vi "PicoScope4000aGetBlock.vi"(8 "Acquisition Settings":T3 {"Down Sample Ratio" min=1 step=1; "Down-Sample Mode" items=["None", "Aggregate", "Decimate", "Average"]}, 9 "Enabled array":i16[](array[numeric]), 10 "handle in":i16, 11 "error in":errorcluster) -> (0 "Min Buffers":T1, 1 "Buffers (Max or non-aggregated)":T2, 2 "handle out":i16, 3 "error out":errorcluster, 4 "overflow":i16, 6 "noOfSamples":u32)   [LabVIEW 2009]
doc: "This VI collects a block of data from the oscilloscope. This can be called in a loop in order to continually collect blocks of data. The oscilloscope should first be set up by using PicoScope3000aSettings.vi. The VI outputs data arrays in two clusters (max and min). If not using aggregation, 'Min Buffers' is not used."
uses:
  ps4000A.dll
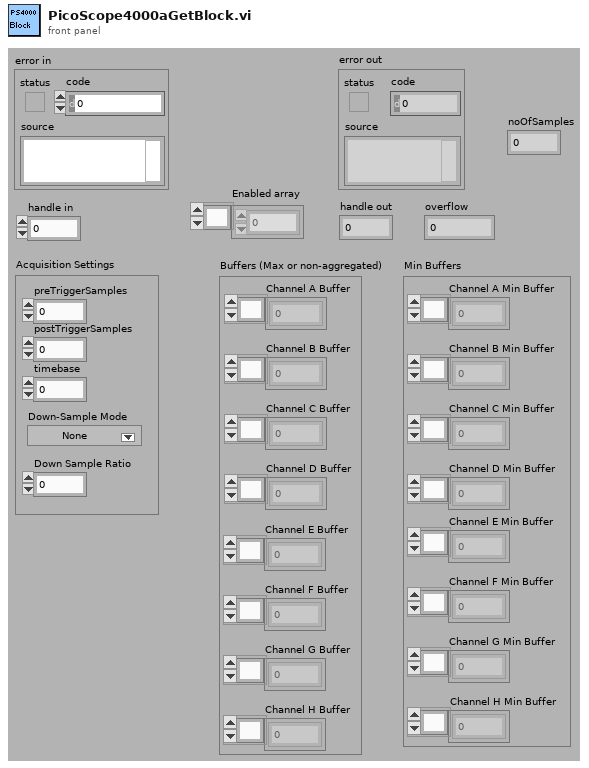
[diagram p1: front panel]
types:
  T1 = cluster{"Channel A Min Buffer":i16[], "Channel B Min Buffer":i16[], "Channel C Min Buffer":i16[], "Channel D Min Buffer":i16[], "Channel E Min Buffer":i16[], "Channel F Min Buffer":i16[], "Channel G Min Buffer":i16[], "Channel H Min Buffer":i16[]}
  T2 = cluster{"Channel D Buffer":i16[], "Channel C Buffer":i16[], "Channel B Buffer":i16[], "Channel A Buffer":i16[], "Channel H Buffer":i16[], "Channel G Buffer":i16[], "Channel F Buffer":i16[], "Channel E Buffer":i16[]}
  T3 = cluster{"preTriggerSamples":i32, "postTriggerSamples":i32, "timebase":u32, "Down-Sample Mode":u32, "Down Sample Ratio":u32}
  T4 = cluster{"Channel A Min Buffer":i16[], "Channel B Min Buffer":i16[], "Channel C Min Buffer":i16[], "Channel D Min Buffer":i16[], "Channel H Min Buffer":i16[], "Channel G Min Buffer":i16[], "Channel F Min Buffer":i16[], "Channel E Min Buffer":i16[]}
  T5 = cluster{"Channel D Buffer":i16[], "Channel C Buffer":i16[], "Channel B Buffer":i16[], "Channel A Buffer":i16[], "Channel E Buffer":i16[], "Channel F Buffer":i16[], "Channel G Buffer":i16[], "Channel H Buffer":i16[]}
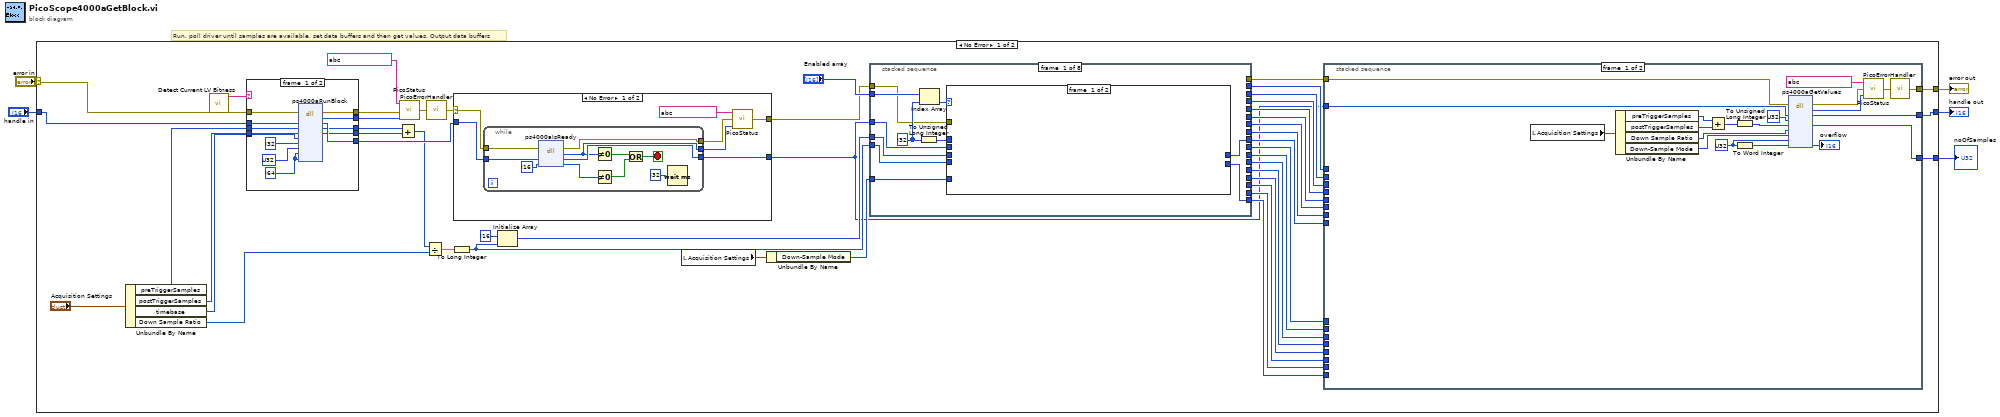
[diagram p0: block diagram]
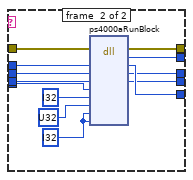
[diagram p2: hidden frame]
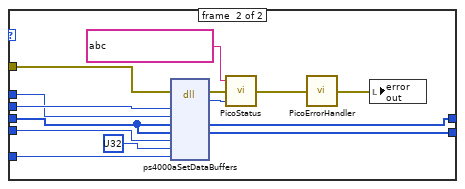
[diagram p3: hidden frame]
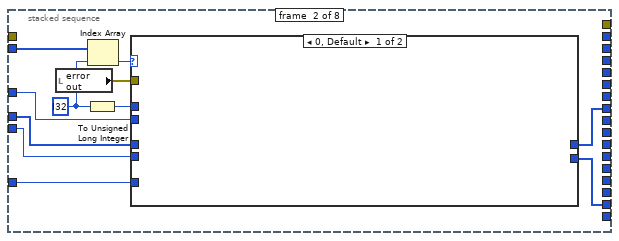
[diagram p4: hidden frame]
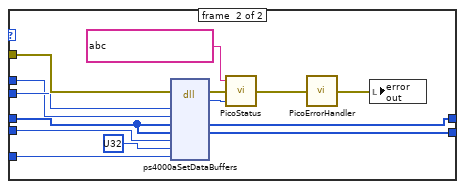
[diagram p5: hidden frame]
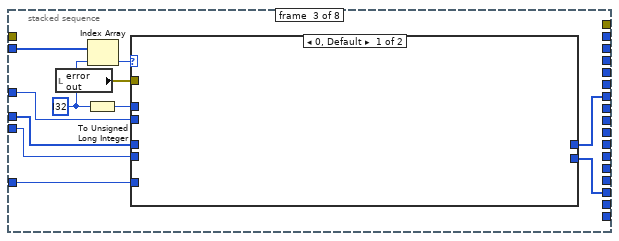
[diagram p6: hidden frame]
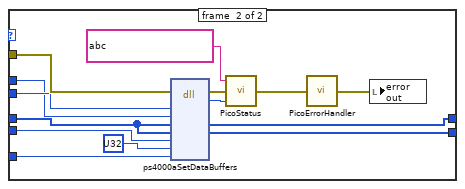
[diagram p7: hidden frame]
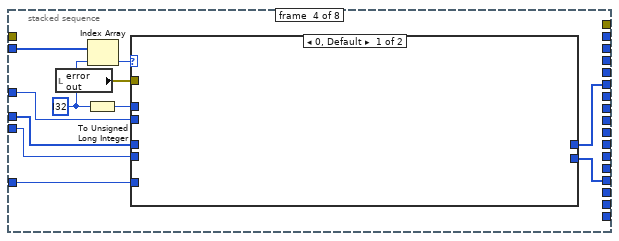
[diagram p8: hidden frame]
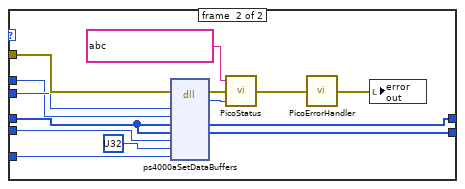
[diagram p9: hidden frame]
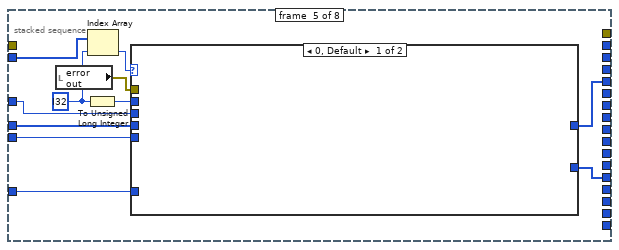
[diagram p10: hidden frame]
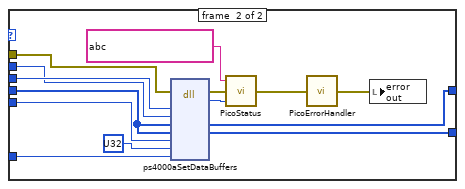
[diagram p11: hidden frame]
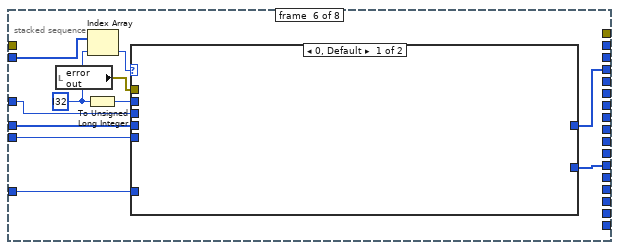
[diagram p12: hidden frame]
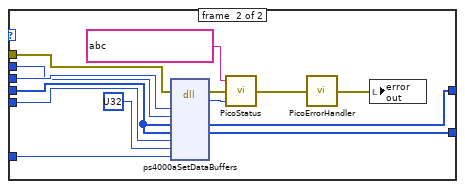
[diagram p13: hidden frame]
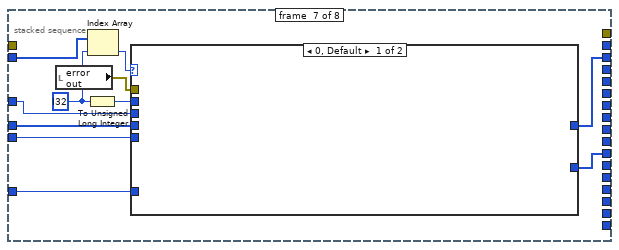
[diagram p14: hidden frame]
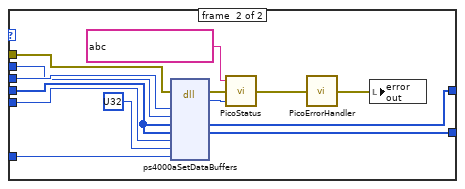
[diagram p15: hidden frame]
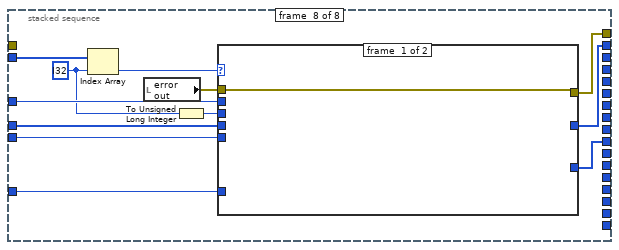
[diagram p16: hidden frame]
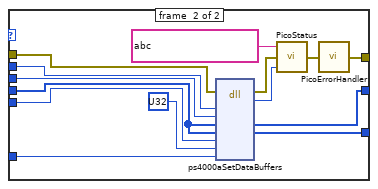
[diagram p17: hidden frame]
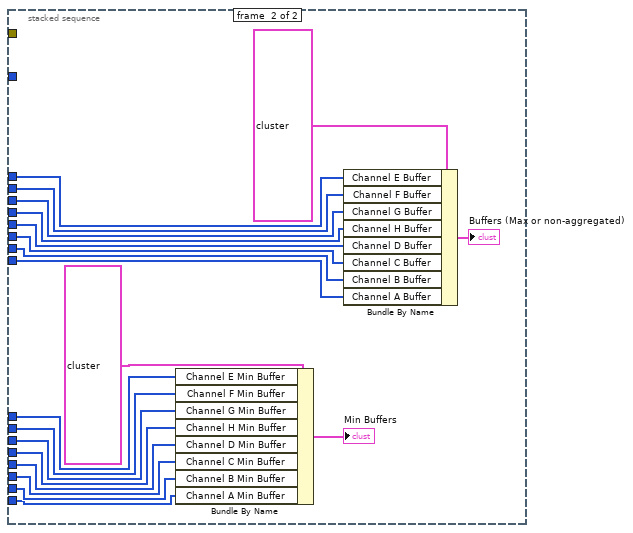
[diagram p18: hidden frame]
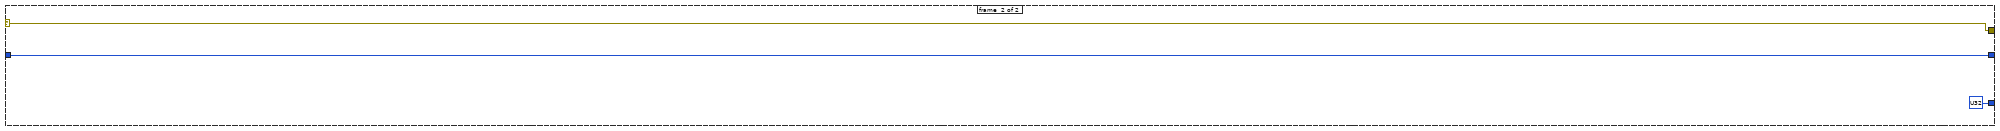
[diagram p20: hidden frame]
diagram:
  # "Run, poll driver until samples are available, set data buffers and then get values. Output data buffers"
  n1 = case shown="No Error" "error in" {
    selector: "error in" -> [w40 w342]
    tunnel: [w41 w342] -> w4
    tunnel: "handle in" -> [w39 w341]
    tunnel: [w38 w341] -> w2
    tunnel: [w7 u32 ? ("noOfSamples")] -> w1
    frame #0 {
      n2 = Unbundle By Name("Acquisition Settings") -> ("preTriggerSamples"=w46:i32, "postTriggerSamples"=w45:i32, "timebase"=w47:u32, "Down Sample Ratio"=w35:u32)
      n3 = call "Detect Current LV Bitness.vi"() -> ("bitness"=w6:string)  [unwired: 11 in]
      n4 = case shown="\"32\", Default" w6 {
        tunnel: [w63 w76] -> w51
        tunnel: [w62 w75] -> w50
        tunnel: [w61 w74] -> w49
        tunnel: w47 -> [w60 w73]
        tunnel: w46 -> [w59 w72]
        tunnel: w45 -> [w58 w71]
        tunnel: [w57 w70] -> w44
        tunnel: [w56 w69] -> w43
        tunnel: w40 -> [w55 w68]
        tunnel: w39 -> [w54 w67]
        frame #0 {
          w53 = i64 ? ("pParameter")
          n5 = dll-call lib="ps4000A.dll" fn="ps4000aRunBlock" ("ps3000.dll:_ps3000_open_unit@0")(error in=w55, "handle"=w54, "preTriggerSamples"=w59, "postTriggerSamples"=w58, "timebase"=w60, "timeindisposed"=i32 ? ("pParameter"), "segmentIndex"=u32 ? ("pParameter"), "lpReady"=w53, "pParameter"=w53) -> (error out=w56:errorcluster, "PICO_STATUS"=w57:u32, "handle"=w63:i16, "preTriggerSamples"=w62:i32, "postTriggerSamples"=w61:i32)  [unwired: 7 in, 1 out]
        }
        frame #1 {
          w65 = i32 ? ("pParameter")
          n6 = dll-call lib="ps4000A.dll" fn="ps4000aRunBlock" ("ps3000.dll:_ps3000_open_unit@0")(error in=w68, "handle"=w67, "preTriggerSamples"=w72, "postTriggerSamples"=w71, "timebase"=w73, "timeindisposed"=i32 ? ("pParameter"), "segmentIndex"=u32 ? ("pParameter"), "lpReady"=w65, "pParameter"=w65) -> (error out=w69:errorcluster, "PICO_STATUS"=w70:u32, "handle"=w76:i16, "preTriggerSamples"=w75:i32, "postTriggerSamples"=w74:i32)  [unwired: 7 in, 1 out]
        }
      }
      n7 = Add(x=w50, y=w49) -> (x+y=w37:i32)
      n8 = call "PicoStatus.vi"("PICO STATUS"=w44, "error in"=w43, "source"=string ?) -> ("error out"=w33:errorcluster)
      n9 = Divide(x=w37, y=w35) -> (x/y=w36:dbl)
      n10 = call "PicoErrorHandler.vi"("error in"=w33) -> ("error out"=w32:errorcluster)
      n11 = To Long Integer(number=w36) -> (32bit integer=w11:i32)
      n12 = case shown="No Error" w32 {
        selector: w32 -> [w324 w338]
        tunnel: w51 -> [w326 w339]
        tunnel: [w325 w339] -> w10
        tunnel: [w323 w338] -> w9
        frame #0 {
          n13 = while {
            tunnel: [w337] -> w325
            tunnel: w326 -> [w336]
            tunnel: [w331] -> w321
            tunnel: w324 -> [w330]
            tunnel: [w329] -> w322
            stop <- w335 stop-if-true
            n14 = dll-call lib="ps4000A.dll" fn="ps4000aIsReady" ("ps3000.dll:_ps3000_open_unit@0")(error in=w330, "handle"=w336, "ready"=i16 ?) -> (error out=w329:errorcluster, "PICO_STATUS"=w331:u32, "handle"=w337:i16, "ready"=w332:i16)  [unwired: 2 in, 1 out]
            n15 = Not Equal To 0?(x=w331) -> (x != 0?=w333:bool)
            n16 = Not Equal To 0?(x=w332) -> (x != 0?=w334:bool)
            n17 = Or(x=w333, y=w334) -> (x .or. y?=w335:bool)
            n18 = Wait (ms)(milliseconds to wait=i32 ?) -> ()  [unwired: 1 out]
          }
          n19 = call "PicoStatus.vi"("PICO STATUS"=w321, "error in"=w322, "source"=string ?) -> ("error out"=w323:errorcluster)
        }
        frame #1 {
        }
      }
      n20 = Initialize Array(i16 ? ("element"), w11) -> (w13:i16[])
      n21 = local read "Acquisition Settings"() -> (w34:T3)
      n22 = Unbundle By Name(w34) -> ("Down-Sample Mode"=w12:u32)
      n23 = stacked-sequence {
        tunnel: [_ _ _ _ _ _ _ w256] -> w30
        tunnel: [_ _ _ _ _ _ w230 _] -> w29
        tunnel: [_ _ _ _ _ w204 _ _] -> w28
        tunnel: [_ _ _ w155 _ _ _ _] -> w27
        tunnel: [_ _ _ _ w180 _ _ _] -> w26
        tunnel: [_ _ w130 _ _ _ _ _] -> w25
        tunnel: [_ w105 _ _ _ _ _ _] -> w24
        tunnel: [w84 _ _ _ _ _ _ _] -> w23
        tunnel: [_ _ _ _ _ _ _ w255] -> w22
        tunnel: [_ _ _ _ _ _ w229 _] -> w21
        tunnel: [_ _ _ _ _ w205 _ _] -> w20
        tunnel: [_ _ _ _ w179 _ _ _] -> w19
        tunnel: [_ _ _ w154 _ _ _ _] -> w18
        tunnel: [_ _ w129 _ _ _ _ _] -> w17
        tunnel: [_ w104 _ _ _ _ _ _] -> w16
        tunnel: [w83 _ _ _ _ _ _ _] -> w15
        tunnel: "Enabled array" -> [w88 w113 w138 w163 w188 w213 w238 w264]
        tunnel: w13 -> [w85 w110 w135 w160 w185 w210 w235 w261]
        tunnel: w9 -> [w78 _ _ _ _ _ _ _]
        tunnel: w10 -> [w86 w111 w136 w161 w186 w211 w236 w262]
        tunnel: w12 -> [w82 w109 w134 w159 w184 w209 w234 w260]
        tunnel: w11 -> [w79 w106 w131 w156 w181 w206 w231 w257]
        tunnel: [_ _ _ _ _ _ _ w254] -> w8
        frame #0 {
          w81 = i32 ? ("index")
          n24 = To Unsigned Long Integer(number=w81) -> (unsigned 32bit integer=w80:u32)
          n25 = Index Array(array=w88, index=w81) -> (element=w87:i16)
          n26 = case shown="1" w87 {
            tunnel: w78 -> [_ w99]
            tunnel: w86 -> [_ w98]
            tunnel: w85 -> [_ w95]
            tunnel: [_ w97] -> w84
            tunnel: [_ w96] -> w83
            tunnel: w82 -> [_ w93]
            tunnel: w80 -> [_ w91]
            tunnel: w79 -> [_ w90]
            frame #0 {
            }
            frame #1 {
              n27 = dll-call lib="ps4000a.dll" fn="ps4000aSetDataBuffers" ("ps3000.dll:_ps3000_open_unit@0")(error in=w99, "handle"=w98, "channel"=w91, "bufferMax"=w95, "bufferMin"=w95, "bufferLth"=w90, "segmentIndex"=u32 ?, "mode"=w93) -> (error out=w102:errorcluster, "PICO_STATUS"=w101:u32, "bufferMax"=w97:i16[], "bufferMin"=w96:i16[])  [unwired: 7 in, 1 out]
              n28 = call "PicoStatus.vi"("PICO STATUS"=w101, "error in"=w102, "source"=string ?) -> ("error out"=w94:errorcluster)
              n29 = call "PicoErrorHandler.vi"("error in"=w94) -> ("error out"=w89:errorcluster)
              n30 = local write "error out"(w89) -> ()
            }
          }
        }
        frame #1 {
          w108 = i32 ? ("index")
          n31 = local read "error out"() -> (w103:errorcluster)
          n32 = To Unsigned Long Integer(number=w108) -> (unsigned 32bit integer=w107:u32)
          n33 = Index Array(array=w113, index=w108) -> (element=w112:i16)
          n34 = case shown="0, Default" w112 {
            tunnel: w103 -> [_ w124]
            tunnel: w111 -> [_ w123]
            tunnel: w110 -> [_ w120]
            tunnel: [_ w122] -> w105
            tunnel: [_ w121] -> w104
            tunnel: w109 -> [_ w114]
            tunnel: w107 -> [_ w117]
            tunnel: w106 -> [_ w116]
            frame #0 {
            }
            frame #1 {
              n35 = dll-call lib="ps4000a.dll" fn="ps4000aSetDataBuffers" ("ps3000.dll:_ps3000_open_unit@0")(error in=w124, "handle"=w123, "channel"=w117, "bufferMax"=w120, "bufferMin"=w120, "bufferLth"=w116, "segmentIndex"=u32 ?, "mode"=w114) -> (error out=w127:errorcluster, "PICO_STATUS"=w126:u32, "bufferMax"=w122:i16[], "bufferMin"=w121:i16[])  [unwired: 7 in, 1 out]
              n36 = call "PicoStatus.vi"("PICO STATUS"=w126, "error in"=w127, "source"=string ?) -> ("error out"=w119:errorcluster)
              n37 = call "PicoErrorHandler.vi"("error in"=w119) -> ("error out"=w115:errorcluster)
              n38 = local write "error out"(w115) -> ()
            }
          }
        }
        frame #2 {
          w133 = i32 ? ("index")
          n39 = local read "error out"() -> (w128:errorcluster)
          n40 = To Unsigned Long Integer(number=w133) -> (unsigned 32bit integer=w132:u32)
          n41 = Index Array(array=w138, index=w133) -> (element=w137:i16)
          n42 = case shown="0, Default" w137 {
            tunnel: w128 -> [_ w149]
            tunnel: w136 -> [_ w148]
            tunnel: w135 -> [_ w145]
            tunnel: [_ w147] -> w130
            tunnel: [_ w146] -> w129
            tunnel: w134 -> [_ w143]
            tunnel: w132 -> [_ w141]
            tunnel: w131 -> [_ w140]
            frame #0 {
            }
            frame #1 {
              n43 = dll-call lib="ps4000a.dll" fn="ps4000aSetDataBuffers" ("ps3000.dll:_ps3000_open_unit@0")(error in=w149, "handle"=w148, "channel"=w141, "bufferMax"=w145, "bufferMin"=w145, "bufferLth"=w140, "segmentIndex"=u32 ?, "mode"=w143) -> (error out=w152:errorcluster, "PICO_STATUS"=w151:u32, "bufferMax"=w147:i16[], "bufferMin"=w146:i16[])  [unwired: 7 in, 1 out]
              n44 = call "PicoStatus.vi"("PICO STATUS"=w151, "error in"=w152, "source"=string ?) -> ("error out"=w144:errorcluster)
              n45 = call "PicoErrorHandler.vi"("error in"=w144) -> ("error out"=w139:errorcluster)
              n46 = local write "error out"(w139) -> ()
            }
          }
        }
        frame #3 {
          w158 = i32 ? ("index")
          n47 = local read "error out"() -> (w153:errorcluster)
          n48 = To Unsigned Long Integer(number=w158) -> (unsigned 32bit integer=w157:u32)
          n49 = Index Array(array=w163, index=w158) -> (element=w162:i16)
          n50 = case shown="0, Default" w162 {
            tunnel: w153 -> [_ w174]
            tunnel: w161 -> [_ w173]
            tunnel: w160 -> [_ w170]
            tunnel: [_ w172] -> w155
            tunnel: [_ w171] -> w154
            tunnel: w159 -> [_ w168]
            tunnel: w157 -> [_ w166]
            tunnel: w156 -> [_ w165]
            frame #0 {
            }
            frame #1 {
              n51 = dll-call lib="ps4000a.dll" fn="ps4000aSetDataBuffers" ("ps3000.dll:_ps3000_open_unit@0")(error in=w174, "handle"=w173, "channel"=w166, "bufferMax"=w170, "bufferMin"=w170, "bufferLth"=w165, "segmentIndex"=u32 ?, "mode"=w168) -> (error out=w177:errorcluster, "PICO_STATUS"=w176:u32, "bufferMax"=w172:i16[], "bufferMin"=w171:i16[])  [unwired: 7 in, 1 out]
              n52 = call "PicoStatus.vi"("PICO STATUS"=w176, "error in"=w177, "source"=string ?) -> ("error out"=w169:errorcluster)
              n53 = call "PicoErrorHandler.vi"("error in"=w169) -> ("error out"=w164:errorcluster)
              n54 = local write "error out"(w164) -> ()
            }
          }
        }
        frame #4 {
          w183 = i32 ? ("index")
          n55 = local read "error out"() -> (w178:errorcluster)
          n56 = To Unsigned Long Integer(number=w183) -> (unsigned 32bit integer=w182:u32)
          n57 = Index Array(array=w188, index=w183) -> (element=w187:i16)
          n58 = case shown="0, Default" w187 {
            tunnel: w178 -> [_ w199]
            tunnel: w186 -> [_ w198]
            tunnel: w185 -> [_ w195]
            tunnel: [_ w197] -> w180
            tunnel: [_ w196] -> w179
            tunnel: w184 -> [_ w193]
            tunnel: w182 -> [_ w191]
            tunnel: w181 -> [_ w190]
            frame #0 {
            }
            frame #1 {
              n59 = dll-call lib="ps4000a.dll" fn="ps4000aSetDataBuffers" ("ps3000.dll:_ps3000_open_unit@0")(error in=w199, "handle"=w198, "channel"=w191, "bufferMax"=w195, "bufferMin"=w195, "bufferLth"=w190, "segmentIndex"=u32 ?, "mode"=w193) -> (error out=w202:errorcluster, "PICO_STATUS"=w201:u32, "bufferMax"=w197:i16[], "bufferMin"=w196:i16[])  [unwired: 7 in, 1 out]
              n60 = call "PicoStatus.vi"("PICO STATUS"=w201, "error in"=w202, "source"=string ?) -> ("error out"=w194:errorcluster)
              n61 = call "PicoErrorHandler.vi"("error in"=w194) -> ("error out"=w189:errorcluster)
              n62 = local write "error out"(w189) -> ()
            }
          }
        }
        frame #5 {
          w208 = i32 ? ("index")
          n63 = local read "error out"() -> (w203:errorcluster)
          n64 = To Unsigned Long Integer(number=w208) -> (unsigned 32bit integer=w207:u32)
          n65 = Index Array(array=w213, index=w208) -> (element=w212:i16)
          n66 = case shown="0, Default" w212 {
            tunnel: w203 -> [_ w224]
            tunnel: w211 -> [_ w223]
            tunnel: w210 -> [_ w220]
            tunnel: [_ w222] -> w204
            tunnel: [_ w221] -> w205
            tunnel: w209 -> [_ w218]
            tunnel: w207 -> [_ w216]
            tunnel: w206 -> [_ w215]
            frame #0 {
            }
            frame #1 {
              n67 = dll-call lib="ps4000a.dll" fn="ps4000aSetDataBuffers" ("ps3000.dll:_ps3000_open_unit@0")(error in=w224, "handle"=w223, "channel"=w216, "bufferMax"=w220, "bufferMin"=w220, "bufferLth"=w215, "segmentIndex"=u32 ?, "mode"=w218) -> (error out=w227:errorcluster, "PICO_STATUS"=w226:u32, "bufferMax"=w222:i16[], "bufferMin"=w221:i16[])  [unwired: 7 in, 1 out]
              n68 = call "PicoStatus.vi"("PICO STATUS"=w226, "error in"=w227, "source"=string ?) -> ("error out"=w219:errorcluster)
              n69 = call "PicoErrorHandler.vi"("error in"=w219) -> ("error out"=w214:errorcluster)
              n70 = local write "error out"(w214) -> ()
            }
          }
        }
        frame #6 {
          w233 = i32 ? ("index")
          n71 = local read "error out"() -> (w228:errorcluster)
          n72 = To Unsigned Long Integer(number=w233) -> (unsigned 32bit integer=w232:u32)
          n73 = Index Array(array=w238, index=w233) -> (element=w237:i16)
          n74 = case shown="0, Default" w237 {
            tunnel: w228 -> [_ w249]
            tunnel: w236 -> [_ w248]
            tunnel: w235 -> [_ w245]
            tunnel: [_ w247] -> w230
            tunnel: [_ w246] -> w229
            tunnel: w234 -> [_ w243]
            tunnel: w232 -> [_ w241]
            tunnel: w231 -> [_ w240]
            frame #0 {
            }
            frame #1 {
              n75 = dll-call lib="ps4000a.dll" fn="ps4000aSetDataBuffers" ("ps3000.dll:_ps3000_open_unit@0")(error in=w249, "handle"=w248, "channel"=w241, "bufferMax"=w245, "bufferMin"=w245, "bufferLth"=w240, "segmentIndex"=u32 ?, "mode"=w243) -> (error out=w252:errorcluster, "PICO_STATUS"=w251:u32, "bufferMax"=w247:i16[], "bufferMin"=w246:i16[])  [unwired: 7 in, 1 out]
              n76 = call "PicoStatus.vi"("PICO STATUS"=w251, "error in"=w252, "source"=string ?) -> ("error out"=w244:errorcluster)
              n77 = call "PicoErrorHandler.vi"("error in"=w244) -> ("error out"=w239:errorcluster)
              n78 = local write "error out"(w239) -> ()
            }
          }
        }
        frame #7 {
          w259 = i32 ? ("index")
          n79 = Index Array(array=w264, index=w259) -> (element=w263:i16)
          n80 = local read "error out"() -> (w253:errorcluster)
          n81 = To Unsigned Long Integer(number=w259) -> (unsigned 32bit integer=w258:u32)
          n82 = case shown="1" w263 {
            tunnel: w253 -> [w265 w276]
            tunnel: w262 -> [_ w275]
            tunnel: w261 -> [_ w272]
            tunnel: [_ w274] -> w256
            tunnel: [_ w273] -> w255
            tunnel: w260 -> [_ w270]
            tunnel: w258 -> [_ w268]
            tunnel: w257 -> [_ w267]
            tunnel: [w265 w266] -> w254
            frame #0 {
            }
            frame #1 {
              n83 = dll-call lib="ps4000a.dll" fn="ps4000aSetDataBuffers" ("ps3000.dll:_ps3000_open_unit@0")(error in=w276, "handle"=w275, "channel"=w268, "bufferMax"=w272, "bufferMin"=w272, "bufferLth"=w267, "segmentIndex"=u32 ?, "mode"=w270) -> (error out=w279:errorcluster, "PICO_STATUS"=w278:u32, "bufferMax"=w274:i16[], "bufferMin"=w273:i16[])  [unwired: 7 in, 1 out]
              n84 = call "PicoStatus.vi"("PICO STATUS"=w278, "error in"=w279, "source"=string ?) -> ("error out"=w271:errorcluster)
              n85 = call "PicoErrorHandler.vi"("error in"=w271) -> ("error out"=w266:errorcluster)
            }
          }
        }
      }
      n86 = stacked-sequence {
        tunnel: w10 -> [w299 _]
        tunnel: [w292 _] -> w41
        tunnel: [w291 _] -> w38
        tunnel: w27 -> [_ w317]
        tunnel: w25 -> [_ w318]
        tunnel: w24 -> [_ w319]
        tunnel: w23 -> [_ w316]
        tunnel: w8 -> [w283 _]
        tunnel: w26 -> [_ w315]
        tunnel: w28 -> [_ w314]
        tunnel: w30 -> [_ w313]
        tunnel: w29 -> [_ w312]
        tunnel: w22 -> [_ w307]
        tunnel: w21 -> [_ w306]
        tunnel: w20 -> [_ w305]
        tunnel: w19 -> [_ w304]
        tunnel: w18 -> [_ w303]
        tunnel: w17 -> [_ w302]
        tunnel: w16 -> [_ w301]
        tunnel: w15 -> [_ w300]
        tunnel: [w280 _] -> w7
        frame #0 {
          w297 = u32 ? ("overflow")
          n87 = local read "Acquisition Settings"() -> (w289:T3)
          n88 = Unbundle By Name(w289) -> ("preTriggerSamples"=w286:i32, "postTriggerSamples"=w287:i32, "Down Sample Ratio"=w288:u32, "Down-Sample Mode"=w284:u32)
          n89 = Add(x=w286, y=w287) -> (x+y=w285:i32)
          n90 = To Unsigned Long Integer(number=w285) -> (unsigned 32bit integer=w282:u32)
          n91 = To Word Integer(number=w297) -> (16bit integer=w281:i16)
          n92 = dll-call lib="ps4000a.dll" fn="ps4000aGetValues" ("ps3000.dll:_ps3000_open_unit@0")(error in=w283, "handle"=w299, "startIndex"=u32 ?, "noOfSamples"=w282, "downSampleRatio"=w288, "downSampleRatioMode"=w284, "segmentIndex"=w297, "overflow"=w281) -> (error out=w295:errorcluster, "PICO_STATUS"=w296:u32, "handle"=w291:i16, "noOfSamples"=w280:u32, "overflow"=→"overflow":i16)  [unwired: 6 in, 1 out]
          n93 = call "PicoStatus.vi"("PICO STATUS"=w296, "error in"=w295, "source"=string ?) -> ("error out"=w293:errorcluster)
          n94 = call "PicoErrorHandler.vi"("error in"=w293) -> ("error out"=w292:errorcluster)
        }
        frame #1 {
          n95 = Bundle By Name(cluster=T4 ? ("Min Buffers"), "Channel E Min Buffer"=w307, "Channel F Min Buffer"=w306, "Channel G Min Buffer"=w305, "Channel H Min Buffer"=w304, "Channel D Min Buffer"=w303, "Channel C Min Buffer"=w302, "Channel B Min Buffer"=w301, "Channel A Min Buffer"=w300) -> (→"Min Buffers":T4)
          n96 = Bundle By Name(cluster=T5 ? ("Buffers (Max or non-aggregated)"), "Channel E Buffer"=w313, "Channel F Buffer"=w312, "Channel G Buffer"=w314, "Channel H Buffer"=w315, "Channel D Buffer"=w317, "Channel C Buffer"=w318, "Channel B Buffer"=w319, "Channel A Buffer"=w316) -> (→"Buffers (Max or non-aggregated)":T5)
        }
      }
    }
    frame #1 {
    }
  }
  "error out" <- w4
  "handle out" <- w2
  "noOfSamples" <- w1
